vi "AG34405 Configure DC Current.vi"(0 "VISA resource name":refnum<visa-resource-name>, 5 "Range (6:Auto)":T2(ring)=enum."Auto", 7 "Resolution (5:Default)":T1(ring)=enum."Default", 11 "error in (no error)":errorcluster) -> (4 "VISA resource name out":refnum<visa-resource-name>, 15 "error out":errorcluster)   [LabVIEW 2018]
doc: "This VI allows you to control various settings for performing DC Current measurements. You can independently control the range and resolution."
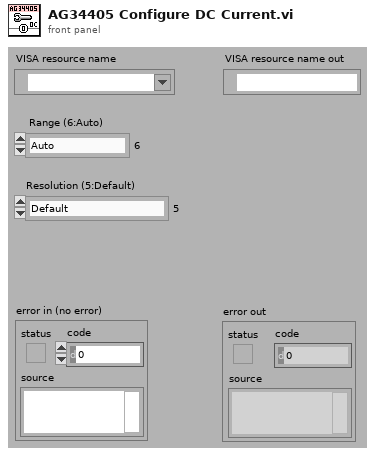
[diagram p1: front panel]
types:
  T1 = enum16{"4 1/2", "5 1/2", "6 1/2", "Least", "Highest", "Default"}
  T2 = enum16{"100 uA", "1 mA", "10 mA", "100 mA", "1 A", "3 A", "Auto", "Minimum", "Maximum", "Default"}
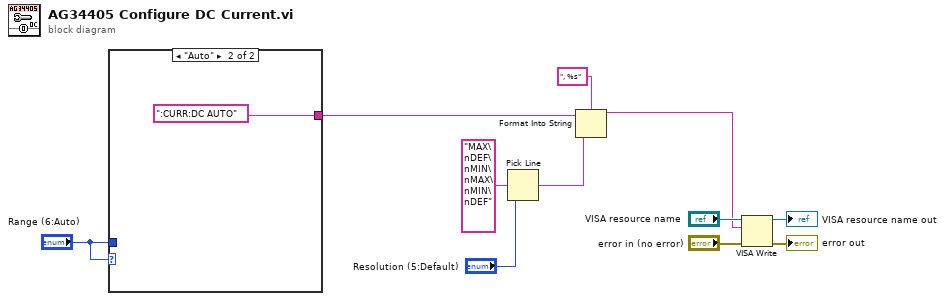
[diagram p0: block diagram]
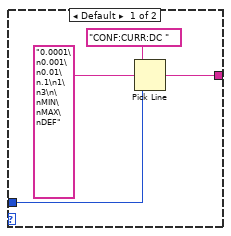
[diagram p2: hidden frame]
diagram:
  n1 = case shown="\"Auto\"" "Range (6:Auto)" {
    tunnel: "Range (6:Auto)" -> [w14 _]
    tunnel: [w13 ":CURR:DC AUTO"] -> w1
    frame Default {
      n2 = Pick Line(string ("")="CONF:CURR:DC ", multi-line string="0.0001\n0.001\n0.01\n.1\n1\n3\n\nMIN\nMAX\nDEF", line index=w14) -> (output string=w13:string)
    }
    frame "Auto" {
    }
  }
  n3 = Pick Line(multi-line string="MAX\nDEF\nMIN\nMAX\nMIN\nDEF", line index="Resolution (5:Default)") -> (output string=w4:string)  [unwired: 1 in]
  n4 = Format Into String(format string=", %s", initial string=w1, w4) -> (resulting string=w3:string)  [unwired: 1 in, 1 out]
  n5 = VISA Write(VISA resource name="VISA resource name", write buffer=w3, error in (no error)="error in (no error)") -> (VISA resource name out=→"VISA resource name out":refnum<visa-resource-name>, error out=→"error out":errorcluster)  [unwired: 1 out]
